vi "IncrementCellPos.vi"(8 "error in (no error)":errorcluster, 11 "SnakeBodyCell in":refnum<class "SnakeBodyCell.lvclass">) -> (0 "error out":errorcluster, 3 "SnakeBodyCell out":refnum<class "SnakeBodyCell.lvclass">)   [LabVIEW 2018, in "SnakeBodyCell.lvclass"]
uses:
  SnakeBodyCell.lvclass
  SnakeBodyCell.lvclass/SnakeBodyCell.ctl
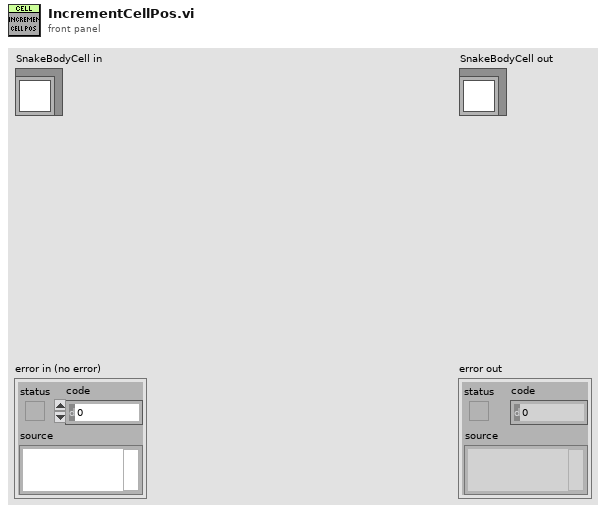
[diagram p1: front panel]
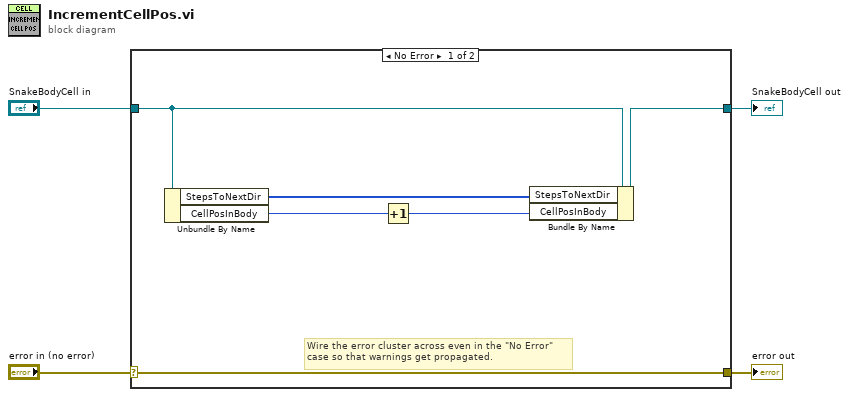
[diagram p0: block diagram]
diagram:
  n1 = case shown="No Error" "error in (no error)" {
    selector: "error in (no error)" -> [w10 w12]
    tunnel: [w10 w12] -> w3
    tunnel: [w8 w11] -> w1
    tunnel: "SnakeBodyCell in" -> [w9 w11]
    frame No Error {
      # "Wire the error cluster across even in the \"No Error\"\ncase so that warnings get propagated."
      n2 = Unbundle By Name(w9) -> ("StepsToNextDir"=w5:u16[], "CellPosInBody"=w7:u16)
      n3 = Increment(x=w7) -> (x+1=w6:u16)
      n4 = Bundle By Name(cluster=w9, "StepsToNextDir"=w5, "CellPosInBody"=w6) -> (w8:refnum<class "SnakeBodyCell.lvclass">)
    }
    frame Error {
    }
  }
  "error out" <- w3
  "SnakeBodyCell out" <- w1
